vi "custom stimulus old.vi"() -> ()   [LabVIEW 2014]
uses:
  <vilib>/userdefined/High Color/IMAQdx.ctl
  <vilib>/Utility/file.llb/Write To Spreadsheet File (DBL).vi
  <vilib>/Utility/file.llb/Write To Spreadsheet File (string).vi
  <vilib>/Utility/file.llb/Read From Spreadsheet File (DBL).vi
  <vilib>/vision/driver/NI_Vision_Acquisition_Software.lvlib
panel:
  in  "Wait before recording (s)":dbl
  in  "Tags":string
  in  "Wait between stimuli (frames)":i32
  in  "Trials Per Power":i32
  in  "Start Recording":bool
  in  "Average Power":dbl
  in  "Frames":i32
  out "Error":string
  out "Save Directory":path
  out "Buffer Number Out":u32
  out "Image":T1(plugin-control)
  in  "stop":bool
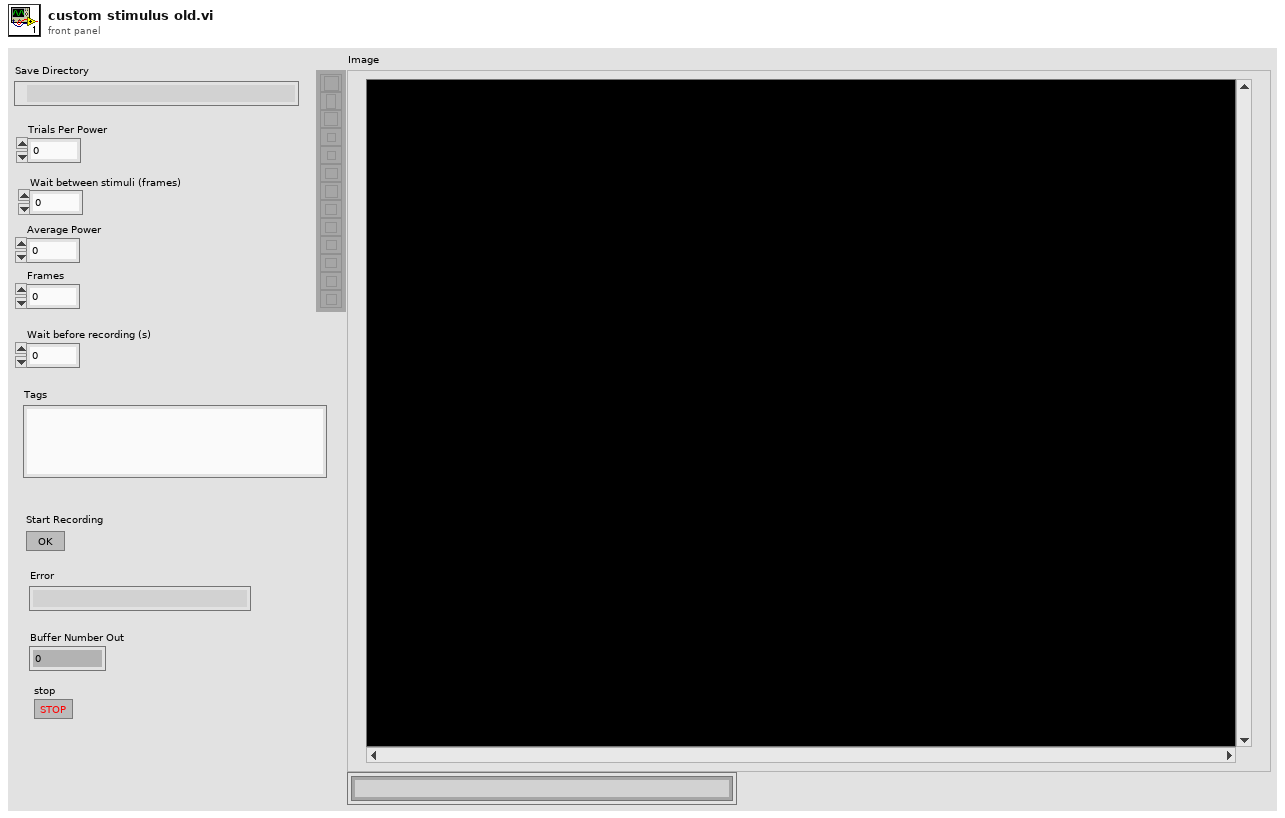
[diagram p1: front panel]
types:
  T1 = typedef "IMAQ Image.ctl" = refnum<image>
  T2 = typedef "IMAQdx.ctl" = refnum<k21>
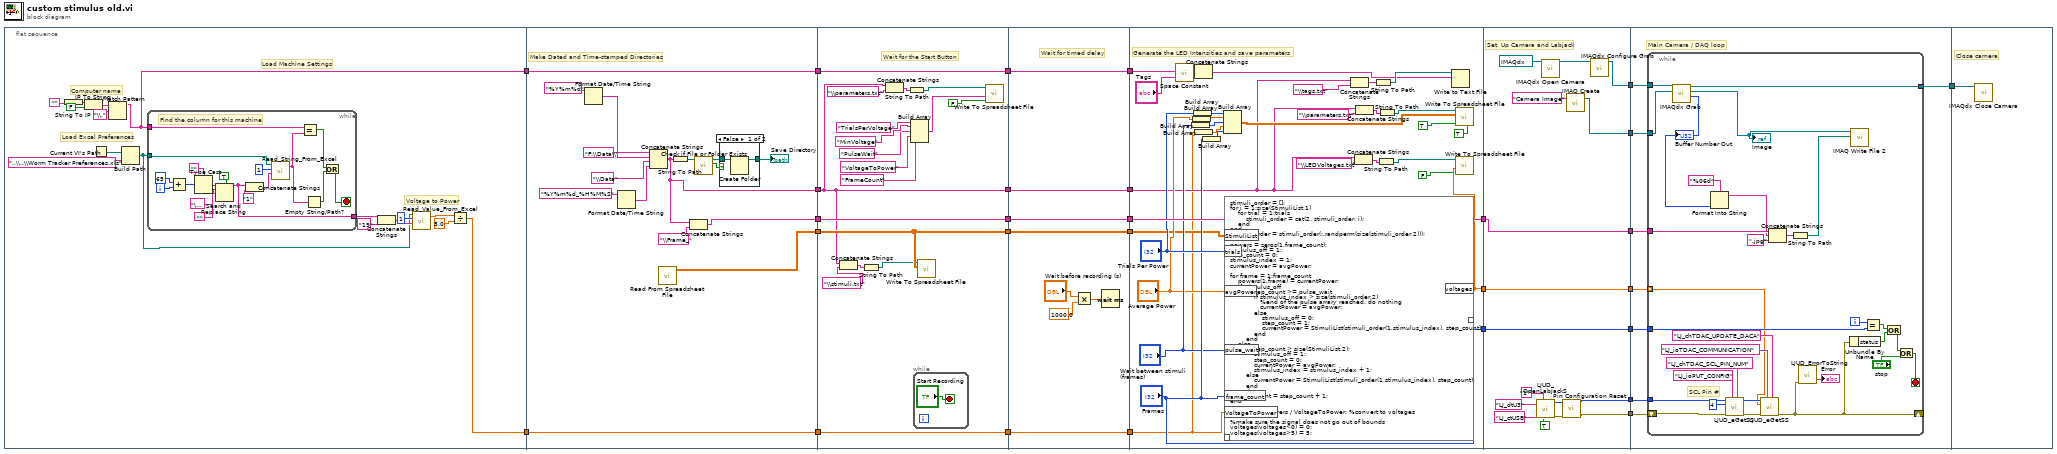
[diagram p0: block diagram]
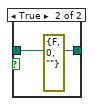
[diagram p2: hidden frame]
diagram:
  n1 = flat-sequence {
    tunnel: [w30] -> w13
    tunnel: [w29] -> w1
    tunnel: [w68] -> w17
    tunnel: [w66] -> w16
    tunnel: [w65] -> w15
    tunnel: [w64] -> w14
    tunnel: w13 -> [w64]
    tunnel: [w63] -> w2
    tunnel: w1 -> [w63]
    tunnel: w17 -> [w99]
    tunnel: [w99] -> w12
    tunnel: w16 -> [w89]
    tunnel: [w89] -> w10
    tunnel: [w91] -> w8
    tunnel: w15 -> [w91]
    tunnel: [w85] -> w6
    tunnel: w14 -> [w85]
    tunnel: [w84] -> w3
    tunnel: w2 -> [w84]
    tunnel: w12 -> [w108]
    tunnel: [w108] -> w11
    tunnel: w10 -> [w107]
    tunnel: [w107] -> w9
    tunnel: w8 -> [w106]
    tunnel: [w106] -> w7
    tunnel: w6 -> [w105]
    tunnel: [w105] -> w5
    tunnel: [w101] -> w4
    tunnel: w3 -> [w101]
    tunnel: w11 -> [w137]
    tunnel: [w137] -> w22
    tunnel: [w135] -> w20
    tunnel: ["Frames"] -> w19
    tunnel: w9 -> [w112]
    tunnel: w7 -> [w121]
    tunnel: w5 -> [w113]
    tunnel: w4 -> [w110]
    tunnel: w22 -> [w150]
    tunnel: [w152] -> w28
    tunnel: [w151] -> w27
    tunnel: [w150] -> w26
    tunnel: [w141] -> w24
    tunnel: [w140] -> w23
    tunnel: [w149] -> w21
    tunnel: w20 -> [w149]
    tunnel: w19 -> [w148]
    tunnel: [w148] -> w18
    tunnel: w28 -> [w163]
    tunnel: w27 -> [w162]
    tunnel: w26 -> [w161]
    tunnel: [w160] -> w25
    tunnel: w24 -> [w159]
    tunnel: w23 -> [w158]
    tunnel: w21 -> [w157]
    tunnel: w18 -> [w156]
    tunnel: w25 -> [w194]
    frame #0 {
      # "Voltage to Power"
      # "Load Excel Preferences"
      # "Computer name"
      # "Load Machine Settings"
      n2 = String To IP(1:"") -> (0:w44:u32)
      n3 = IP To String(1:FALSE, 2:w44) -> (0:w41:string)
      n4 = Current VI's Path() -> (path=w39:path)
      n5 = Match Pattern(string=w41, regular expression="\\.") -> (before substring=w30:string)  [unwired: 1 in, 3 out]
      n6 = Build Path(base path=w39, name or relative path="..\\..\\Worm Tracker Preferences.xls") -> (appended path=w33:path)
      n7 = while {
        tunnel: w33 -> [w57]
        tunnel: w30 -> [w54]
        tunnel: [w45] -> w37
        i -> [w62]
        stop <- w51 stop-if-true
        # "Find the column for this machine"
        n8 = Add(x=65, y=w62) -> (x+y=w60:i32)
        n9 = Type Cast(type="", x=w60) -> (*(type *) &x=w46:string)
        n10 = Search and Replace String(replace all?=TRUE, input string=w46, search string="\u0000", replace string="") -> (result string=w45:string)  [unwired: 4 in, 3 out]
        n11 = Concatenate Strings(w45, "1") -> (w56:string)
        n12 = call "Read_String_From_Excel.vi"("Selected Cell"=w56, "Work Sheet"=1, "Excel File Path"=w57) -> ("Data from Cell"=w55:string)  [unwired: 1 in, 1 out]
        n13 = Equal?(x=w54, y=w55) -> (x = y?=w53:bool)
        n14 = Empty String/Path?(string/path=w55) -> (empty?=w52:bool)
        n15 = Or(x=w53, y=w52) -> (x .or. y?=w51:bool)
      }
      n16 = Concatenate Strings(w37, "19") -> (w35:string)
      n17 = call "Read_Value_From_Excel.vi"("Selected Cell"=w35, "Work Sheet"=1, "Excel File Path"=w33) -> ("Data from Cell"=w32:dbl)  [unwired: 1 in, 1 out]
      n18 = Divide(x=w32, y=5.0) -> (x/y=w29:dbl)
    }
    frame #1 {
      # "Make Dated and Time-stamped Directories"
      n19 = Format Date/Time String(time format string (%c)="%Y%m%d") -> (date/time string=w69:string)  [unwired: 2 in]
      n20 = Format Date/Time String(time format string (%c)="%Y%m%d_%H%M%S") -> (date/time string=w73:string)  [unwired: 2 in]
      n21 = Concatenate Strings("F:\\Data\\", w69, "\\Data", w73) -> (w66:string)
      n22 = call-poly <vilib>:"Read From Spreadsheet File.vi"() -> ("all rows"=w65:dbl[][])  [unwired: 7 in, 4 out]
      n23 = String To Path(string=w66) -> (path=w72:path)
      n24 = Concatenate Strings(w66, "\\Frame_") -> (w68:string)
      n25 = call <vilib>:"Check if File or Folder Exists.vi"("path"=w72) -> ("file or folder exists?"=w77:bool, "dup path"=w76:path)  [unwired: 8 in, 1 out]
      n26 = case shown="False" w77 {
        tunnel: [w79 w81] -> w71
        tunnel: w76 -> [w80 w81]
        frame False {
          n27 = Create Folder(path (use dialog)=w80) -> (created path=w79:path)  [unwired: 2 in, 2 out]
        }
        frame True {
          (unwired) errorcluster {"status"=FALSE, "code"=0, "source"=""} ("error out")
        }
      }
      "Save Directory" <- w71
    }
    frame #2 {
      # "Wait for the Start Button"
      n28 = Concatenate Strings(w89, "\\stimuli.txt") -> (w90:string)
      n29 = String To Path(string=w90) -> (path=w87:path)
      n30 = Concatenate Strings(w89, "\\parameters.txt") -> (w98:string)
      n31 = String To Path(string=w98) -> (path=w97:path)
      n32 = Build Array("TrialsPerVoltage", "MinVoltage", "PulseWait", "VoltageToPower", "FrameCount") -> (w94:string[])
      n33 = while {
        stop <- "Start Recording" stop-if-true
      }
      n34 = call-poly <vilib>:"Write To Spreadsheet File.vi"("2D data"=w91, "file path (dialog if empty)"=w87) -> ()  [unwired: 6 in, 1 out]
      n35 = call-poly <vilib>:"Write To Spreadsheet File.vi"("append to file? (new file:F)"=FALSE, "1D data"=w94, "file path (dialog if empty)"=w97) -> ()  [unwired: 5 in, 1 out]
    }
    frame #3 {
      # "Wait for timed delay"
      n36 = Multiply(x="Wait before recording (s)", y=1000.0) -> (x*y=w103:dbl)
      n37 = Wait (ms)(milliseconds to wait=w103) -> ()  [unwired: 1 out]
    }
    frame #4 {
      # "Generate the LED Intensities and save parameters"
      n38 = call <vilib>:"Space Constant.vi"() -> ("String"=w115:string)
      n39 = Build Array("Wait between stimuli (frames)") -> (w120:i32[])
      n40 = Build Array("Average Power") -> (w122:dbl[])
      n41 = Build Array("Trials Per Power") -> (w128:i32[])
      n42 = Concatenate Strings(w113, w115, "Tags") -> (w114:string)
      n43 = Build Array(w110) -> (w109:dbl[])
      n44 = Build Array("Frames") -> (w111:i32[])
      n45 = Build Array(w128, w122, w120, w109, w111) -> (w126:dbl[][])
      n46 = script code="stimuli_order = [];\nfor i = 1:size(StimuliList,1)\n    for trial = 1:trials\n        stimuli_order = cat(2, stimuli_order, i);\n    end\nend\nstimuli_order = stimuli_order(:,randperm(size(stimuli_order,2)));\n\npowers = zeros(1,frame_count);\nstimulus_off = 1;\nstep_count = 0;\nstimulus_index = 1;\ncurrentPower = avgPower;\n\nfor frame = 1:frame_count\n    powers(1,frame) = currentPower;\n    if stimulus_off\n        if step_count >= pulse_wait\n            if stimulus_index > size(stimuli_order,2)\n               %end of the pulse arrary reached, do nothing\n               currentPower = avgPower;\n            else\n                stimulus_off = 0;\n                step_count = 1;\n                currentPower = StimuliList(stimuli_order(1,stimulus_index), step_count);\n            end\n        end\n    else\n        if step_count > size(StimuliList,2);\n            stimulus_off = 1;\n            step_count = 0;\n            currentPower = avgPower;\n            stimulus_index = stimulus_index + 1;\n        else\n            currentPower = StimuliList(stimuli_order(1,stimulus_index), step_count);\n        end\n    end\n    step_count = step_count + 1;\nend\n\nvoltages = powers / VoltageToPower; %convert to voltages\n\n%make sure the signal does not go out of bounds\nvoltages(voltages<0) = 0;\nvoltages(voltages>5) = 5;"("frame_count"="Frames", "trials"="Trials Per Power", "avgPower"="Average Power", "StimuliList"=w121, "pulse_wait"="Wait between stimuli (frames)", "VoltageToPower"=w110) -> ("voltages"=w135:dbl[])  [unwired: 1 in, 1 out]
      n47 = Concatenate Strings(w112, "\\tags.txt") -> (w118:string)
      n48 = Concatenate Strings(w112, "\\LEDVoltages.txt") -> (w139:string)
      n49 = Concatenate Strings(w112, "\\parameters.txt") -> (w133:string)
      n50 = String To Path(string=w118) -> (path=w117:path)
      n51 = String To Path(string=w139) -> (path=w138:path)
      n52 = String To Path(string=w133) -> (path=w132:path)
      n53 = Write to Text File(file (use dialog)=w117, text=w114) -> ()  [unwired: 2 in, 3 out]
      n54 = call-poly <vilib>:"Write To Spreadsheet File.vi"("append to file? (new file:F)"=FALSE, "1D data"=w135, "file path (dialog if empty)"=w138) -> ()  [unwired: 5 in, 1 out]
      n55 = call-poly <vilib>:"Write To Spreadsheet File.vi"("transpose? (no:F)"=TRUE, "append to file? (new file:F)"=TRUE, "2D data"=w126, "file path (dialog if empty)"=w132) -> ()  [unwired: 4 in, 1 out]
    }
    frame #5 {
      # "Set  Up Camera and Labjack"
      n56 = call "LJUD_OpenLabJackS.vi"("FirstFound"=TRUE, "Address"="1" ("DeviceType"), "ConnectionType"="LJ_ctUSB", "DeviceType"="LJ_dtU3") -> ("error out"=w142:errorcluster, "Handle"=w143:i32)  [unwired: 5 in, 1 out]
      n57 = call <vilib>:"IMAQdx Open Camera.vi"("Session In"=T2 "cam0") -> ("Session Out"=w154:T2)  [unwired: 9 in, 1 out]
      n58 = call "Pin Configuration Reset.vi"("error in"=w142, "Handle In"=w143) -> ("error out"=w140:errorcluster, "Handle Out"=w141:i32)  [unwired: 8 in]
      n59 = call "IMAQ Create"("Image Name"="Camera Image") -> ("New Image"=w151:T1)  [unwired: 4 in, 1 out]
      n60 = call <vilib>:"IMAQdx Configure Grab.vi"("Session In"=w154) -> ("Session Out"=w152:T2)  [unwired: 9 in, 1 out]
    }
    frame #6 {
      # "Main Camera / DAQ loop"
      n61 = while {
        tunnel: w163 -> [w193]
        tunnel: [w192] -> w160
        tunnel: w162 -> [w191]
        tunnel: w161 -> [w189]
        tunnel: w159 -> [w165]
        shift-right: [w167] -> _
        shift-left: w158 -> [w166]
        tunnel: w157 -> [w164] mode=indexing
        tunnel: w156 -> [w175]
        i -> [w176]
        stop <- w182 stop-if-true
        # "SCL Pin #"
        n62 = call <vilib>:"IMAQdx Grab.vi"("Image In"=w191, "Session In"=w193) -> ("Buffer Number Out"=w185:u32, "Image Out"=w190:T1, "Session Out"=w192:T2)  [unwired: 6 in, 1 out]
        "Image" <- w190
        "Buffer Number Out" <- w185
        n63 = Format Into String(format string="%06d" ("string"), w185) -> (resulting string=w184:string)  [unwired: 2 in, 1 out]
        n64 = call "LJUD_eGetSS.vi"("Channel"="LJ_chTDAC_SCL_PIN_NUM", "IOType"="LJ_ioPUT_CONFIG", "error in"=w166, "Value Write"=4, "Handle In"=w165) -> ("error out"=w168:errorcluster, "Handle Out"=w171:i32)  [unwired: 4 in, 1 out]
        n65 = call "LJUD_eGetSS.vi"("Channel"="LJ_chTDAC_UPDATE_DACA", "IOType"="LJ_ioTDAC_COMMUNICATION", "error in"=w168, "Value Write"=w164, "Handle In"=w171) -> ("error out"=w167:errorcluster)  [unwired: 4 in, 2 out]
        n66 = Concatenate Strings(w189, w184, ".jpg" ("string")) -> (w187:string)
        n67 = String To Path(string=w187) -> (path=w186:path)
        n68 = call "LJUD_ErrorToString.vi"("error in"=w167) -> ("String"=→"Error":string)  [unwired: 10 in]
        n69 = Unbundle By Name(w167) -> ("status"=w179:bool)
        n70 = call-poly "IMAQ Write File 2"("File Path"=w186, "Image"=w190) -> ()  [unwired: 8 in, 2 out]
        n71 = Equal?(x=w176, y=w175) -> (x = y?=w178:bool)
        n72 = Or(x=w178, y=w179) -> (x .or. y?=w177:bool)
        n73 = Or(x=w177, y="stop") -> (x .or. y?=w182:bool)
      }
    }
    frame #7 {
      # "Close camera"
      n74 = call <vilib>:"IMAQdx Close Camera.vi"("Session In"=w194) -> ()  [unwired: 10 in, 1 out]
    }
  }
